vi "Autonomous.vi"() -> ()   [LabVIEW 2017]
doc: "This VI starts when autonomous period begins, and will automatically be terminated when it ends. You can carry out timed or sensor driven operations directly to I/O or to subsystems without needing to return to the caller."
uses:
  Motion_Profiler_Class-master/MotionProfiles.lvclass
  <vilib>/Rock Robotics/WPI/SafetyOutput/WPI_SafetyOutputConfigMenu.ctl
  fa3d0b00-d70b-4d5b-8447-19f35fb7f60c.vi
  d1af4e31-2977-4334-b470-f567b7f2c4f2.vi
  <vilib>/Rock Robotics/Network Tables/NT Read String.vi
  <vilib>/Rock Robotics/WPI/Utilities/WPI_GetSetVariantRefNum.vi
  <vilib>/Rock Robotics/Network Tables/NT Read Boolean.vi
panel:
  out "Left Motor":T1(graph)
  out "Left Throttle":dbl(graph)
  out "Right Motor":T2(graph)
  out "Right Throttle":dbl(graph)
  out "Right Bottom Buf Count":i32
  out "Left Bottom Buf Count":i32
  out "Right Under Run":bool
  out "Left Under Run":bool
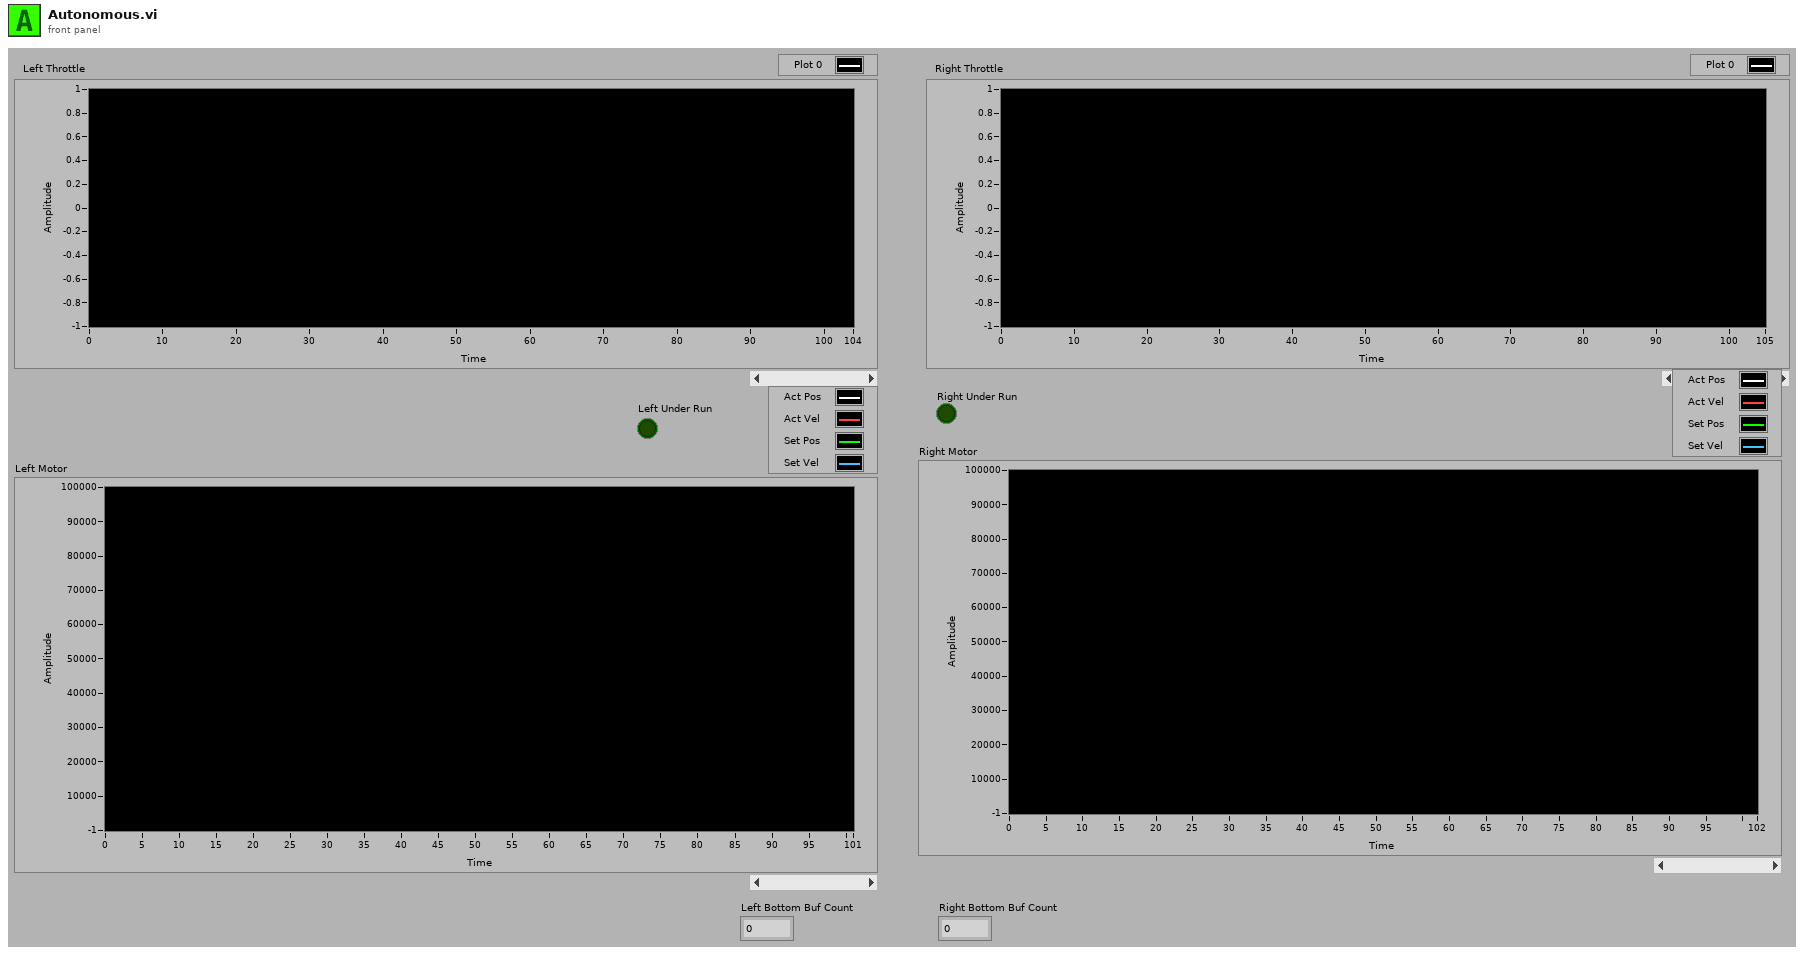
[diagram p1: front panel]
types:
  T1 = cluster{"Set_Pos_(u)":i32, "Set_Pos_(u)":i32, "Act_Vel_(u/100ms)":i32, "Set_Vel_(u/100ms)":i32}
  T2 = cluster{"Set_Vel_(u/100ms)":i32, "Act_Vel_(u/100ms)":i32, "Set_Pos_(u)":i32, "Act_Pos(u)":i32}
  T3 = typedef "WPI_SafetyOutputConfigMenu.ctl" = enum16{"Enable", "Disable"}
  T4 = typedef "WPI_RobotDriveDevRef.ctl" = cluster{"DevStatus":errorcluster, "Motors[]":T5[], "Square Inputs":bool, "Max Output":dbl}
  T5 = typedef "WPI_MotorControlDeviceRef.ctl" = cluster{"DeviceStatus":errorcluster, "Type":T6, "PWM":cluster{"PWM Channel":T7, "DeadBand":T8}, "CAN":cluster{"Device Number":u8, "SetOutput VI Ref":variant, "GetOutput VI Ref":variant, "Enable VI Ref":variant, "Disable VI Ref":variant, "Data":variant}, "Invert":bool, "DIO PWM":cluster{"PWM \"Enable\" Channel":T7, "DIOChannel":T9, "PWM Rate":dbl}}
  T6 = typedef "WPI_MotorControlType.ctl" = enum16{"PWM", "CAN", "DIO PWM"}
  T7 = typedef "FPGA_DIOPWMChannel.ctl" = enum8{"PWM 0", "PWM 1", "PWM 2", "PWM 3", "PWM 4", "PWM 5", "PWM 6", "PWM 7", "PWM 8", "PWM 9", "PWM MXP 0", "PWM MXP 1", "PWM MXP 2", "PWM MXP 3", "PWM MXP 4", "PWM MXP 5", "PWM MXP 6", "PWM MXP 7", "PWM MXP 8", "PWM MXP 9", "Invalid"}
  T8 = typedef "WPI_PWMDeadband.ctl" = cluster{"Name":string, "maxPositivePwm":i32, "minPositivePwm":i32, "centerPwm":i32, "maxNegativePwm":i32, "minNegativePwm":i32, "angularRange":u16}
  T9 = typedef "FPGA_DIOChannel.ctl" = enum8{"DIO 0", "DIO 1", "DIO 2", "DIO 3", "DIO 4", "DIO 5", "DIO 6", "DIO 7", "DIO 8", "DIO 9", "DIO MXP 0", "DIO MXP 1", "DIO MXP 2", "DIO MXP 3", "DIO MXP 4", "DIO MXP 5", "DIO MXP 6", "DIO MXP 7", "DIO MXP 8", "DIO MXP 9", "DIO MXP 10", "DIO MXP 11", "DIO MXP 12", "DIO MXP 13", "DIO MXP 14", "DIO MXP 15", "SPI Port CS1", "SPI Port CS2", "SPI Port CS3", "SPI Port MISO", "SPI Port MOSI", "Invalid"}
  T10 = typedef "MotionProfiles.lvclass/MotionProfile_MP_Class_Status.ctl" = cluster{"Motion Profile Status":cluster{"Top Buffer Remaining":i32, "Top Buffer Count":i32, "Bottom Buffer Count":i32, "Has Underrun?":bool, "Is Underrun?":bool, "Active Point Valid?":bool, "Is Last?":bool, "Profile Slot Select 0":i32, "Output Enable":i32, "Time Duration (ms)":i32, "Profile Slot Select 1":i32}, "TalonState":T11, "MP Is Done":bool, "MP Is Executing":bool, "Set_Vel_(u/100ms)":i32, "Set_Pos_(u)":i32, "Act_Vel_(u/100ms)":i32, "Act_Pos(u)":i32, "Throtle":dbl}
  T11 = typedef "MotionProfiles.lvclass/MotionProfile_TalonSetValueEnum.ctl" = enum16{"Disable", "Enable", "Hold"}
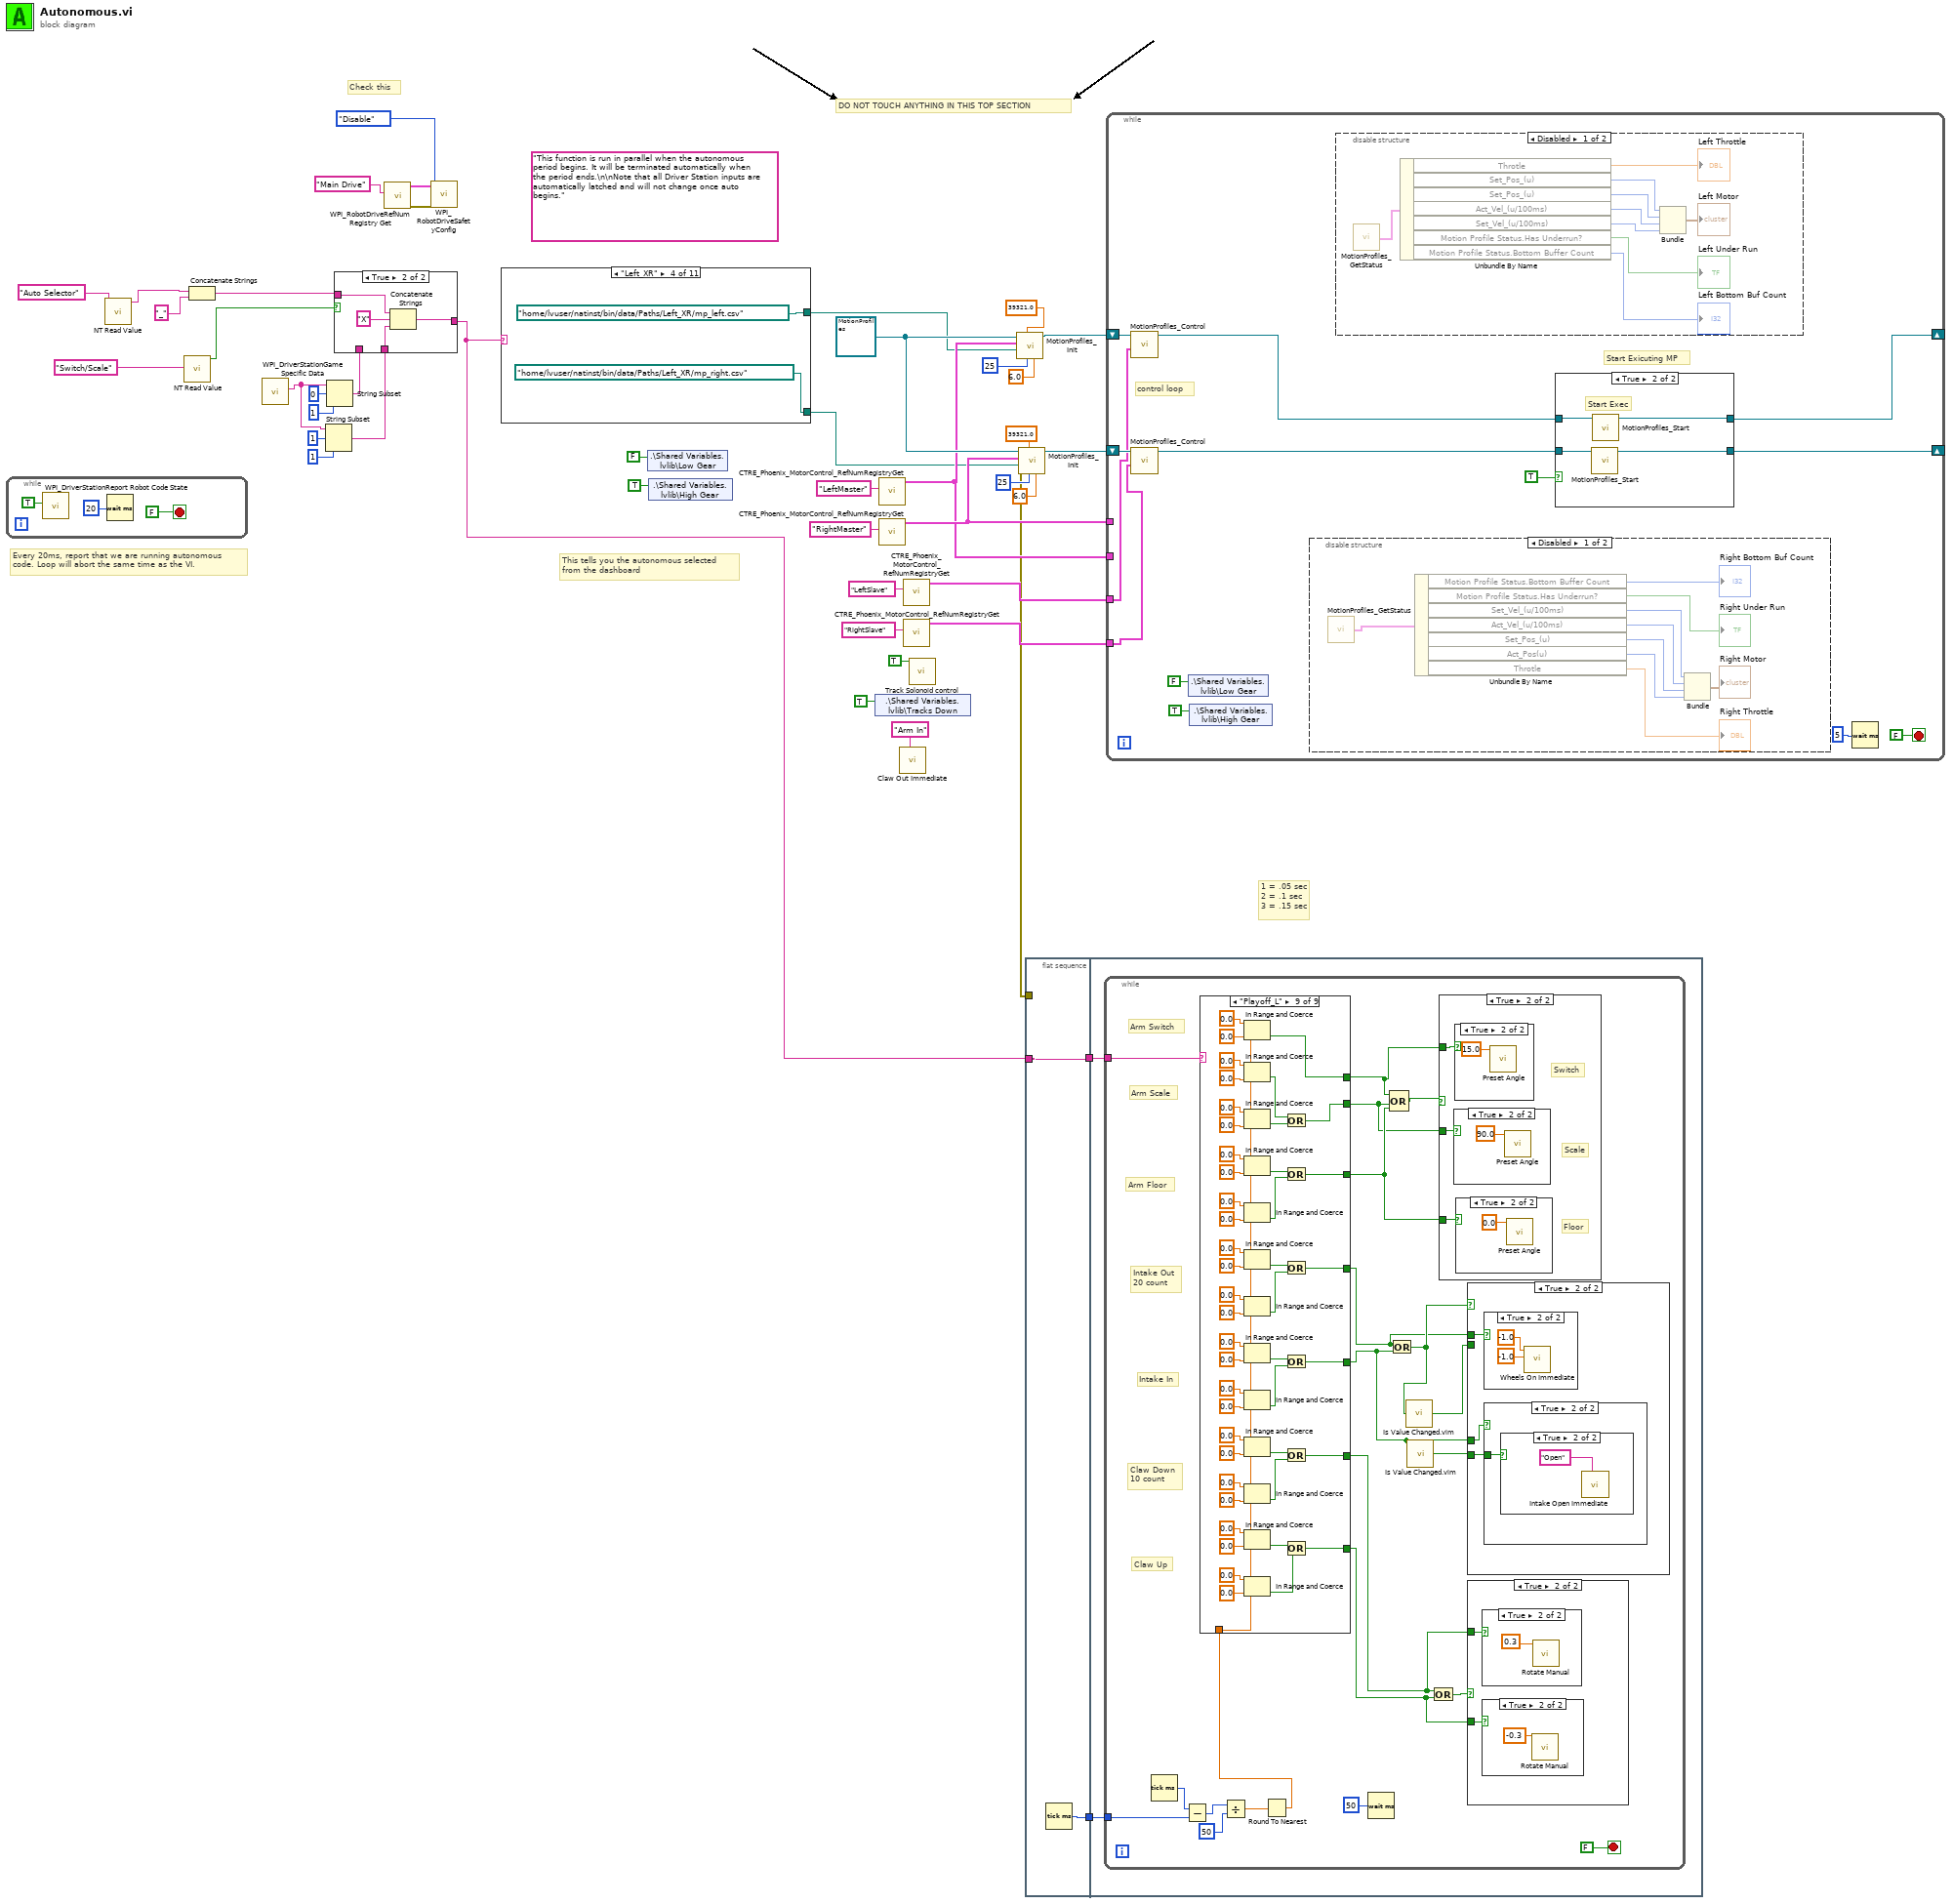
[diagram p0: block diagram]
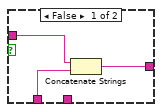
[diagram p2: hidden frame]
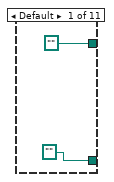
[diagram p3: hidden frame]
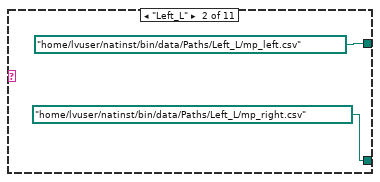
[diagram p4: hidden frame]
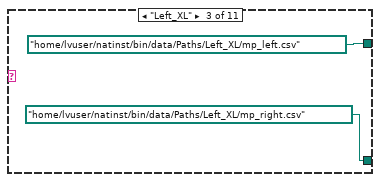
[diagram p5: hidden frame]
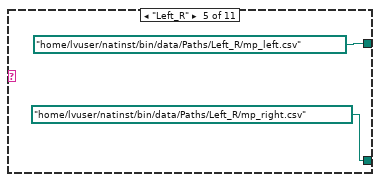
[diagram p6: hidden frame]
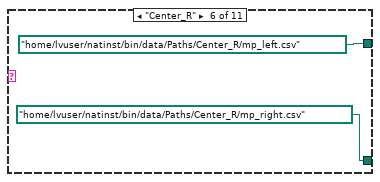
[diagram p7: hidden frame]
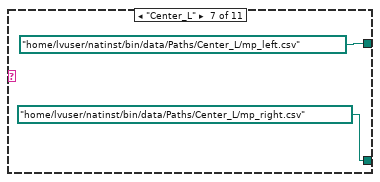
[diagram p8: hidden frame]
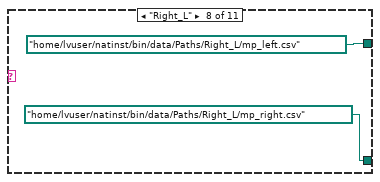
[diagram p9: hidden frame]
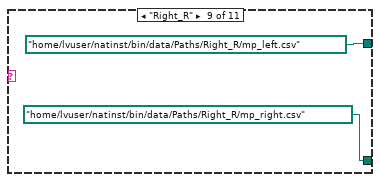
[diagram p10: hidden frame]
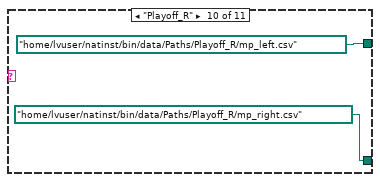
[diagram p11: hidden frame]
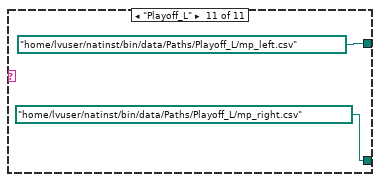
[diagram p12: hidden frame]
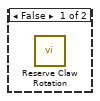
[diagram p13: hidden frame]
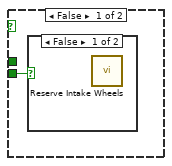
[diagram p16: hidden frame]
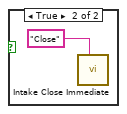
[diagram p17: hidden frame]
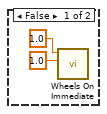
[diagram p20: hidden frame]
diagram:
  w41 = refnum<class "MotionProfiles.lvclass"> refnum ("MotionProfiles.lvclass")
  (unwired) "This function is run in parallel when the autonomous period begins. It will be terminated automatically when the period ends.\n\nNote that all Driver Station inputs are automatically latched and will not change once auto begins."
  # "1 = .05 sec\n2 = .1 sec\n3 = .15 sec"
  # "Check this"
  # "DO NOT TOUCH ANYTHING IN THIS TOP SECTION"
  # "This tells you the autonomous selected\nfrom the dashboard"
  # "Every 20ms, report that we are running autonomous\ncode. Loop will abort the same time as the VI."
  n1 = while {
    stop <- FALSE stop-if-true
    n2 = call <vilib>:"WPI_DriverStationReport Robot Code State.vi"("Autonomous"=TRUE) -> ()  [unwired: 10 in, 1 out]
    n3 = Wait (ms)(milliseconds to wait=u32 20) -> ()  [unwired: 1 out]
  }
  n4 = call-poly <vilib>:"NT Read Value.vi"("Name"="Auto Selector") -> ("String"=w19:string)  [unwired: 9 in, 1 out]
  n5 = call-poly <vilib>:"NT Read Value.vi"("Name"="Switch/Scale") -> ("Boolean"=w2:bool)  [unwired: 9 in, 1 out]
  n6 = Concatenate Strings(w19, "_" ("string")) -> (w6:string)
  n7 = call <vilib>:"WPI_DriverStationGame Specific Data.vi"() -> ("Game Specific Data"=w7:string)  [unwired: 11 in]
  n8 = String Subset(string=w7, offset (0)=1, length (rest)=1 ("length (rest)")) -> (substring=w5:string)
  n9 = String Subset(string=w7, offset (0)=0, length (rest)=1 ("length (rest)")) -> (substring=w4:string)
  n10 = case shown="True" w2 {
    tunnel: w6 -> [w50 w55]
    tunnel: w5 -> [_ w53]
    tunnel: w4 -> [w51 _]
    tunnel: [w49 w52] -> w3
    frame False {
      n11 = Concatenate Strings(w50, w51) -> (w49:string)
    }
    frame True {
      n12 = Concatenate Strings(w55, "X" ("string"), w53) -> (w52:string)
    }
  }
  n13 = call <vilib>:"WPI_RobotDriveRefNum Registry Get.vi"("refnum name"="Main Drive") -> ("error out"=w17:errorcluster, "RobotDriveDevRef"=w16:T4)  [unwired: 9 in]
  n14 = call <vilib>:"WPI_RobotDriveSafetyConfig.vi"("error in (no error)"=w17, "mode"=WPI_SafetyOutputConfigMenu."Disable", "RobotDriveDevRef"=w16) -> ()  [unwired: 7 in, 2 out]
  n15 = case shown="\"Left_XR\"" w3 {
    tunnel: [path "" path "/home/lvuser/natinst/bin/data/Paths/Left_L/mp_right.csv" ("file path (use dialog)") path "/home/lvuser/natinst/bin/data/Paths/Left_XL/mp_right.csv" ("file path (use dialog)") path "/home/lvuser/natinst/bin/data/Paths/Left_XR/mp_right.csv" ("file path (use dialog)") path "/home/lvuser/natinst/bin/data/Paths/Left_R/mp_right.csv" ("file path (use dialog)") path "/home/lvuser/natinst/bin/data/Paths/Center_R/mp_right.csv" ("file path (use dialog)") path "/home/lvuser/natinst/bin/data/Paths/Center_L/mp_right.csv" ("file path (use dialog)") path "/home/lvuser/natinst/bin/data/Paths/Right_L/mp_right.csv" ("file path (use dialog)") path "/home/lvuser/natinst/bin/data/Paths/Right_R/mp_right.csv" ("file path (use dialog)") path "/home/lvuser/natinst/bin/data/Paths/Playoff_R/mp_right.csv" ("file path (use dialog)") path "/home/lvuser/natinst/bin/data/Paths/Playoff_L/mp_right.csv" ("file path (use dialog)")] -> w12
    tunnel: [path "" path "/home/lvuser/natinst/bin/data/Paths/Left_L/mp_left.csv" ("file path (use dialog)") path "/home/lvuser/natinst/bin/data/Paths/Left_XL/mp_left.csv" ("file path (use dialog)") path "/home/lvuser/natinst/bin/data/Paths/Left_XR/mp_left.csv" ("file path (use dialog)") path "/home/lvuser/natinst/bin/data/Paths/Left_R/mp_left.csv" ("file path (use dialog)") path "/home/lvuser/natinst/bin/data/Paths/Center_R/mp_left.csv" ("file path (use dialog)") path "/home/lvuser/natinst/bin/data/Paths/Center_L/mp_left.csv" ("file path (use dialog)") path "/home/lvuser/natinst/bin/data/Paths/Right_L/mp_left.csv" ("file path (use dialog)") path "/home/lvuser/natinst/bin/data/Paths/Right_R/mp_left.csv" ("file path (use dialog)") path "/home/lvuser/natinst/bin/data/Paths/Playoff_R/mp_left.csv" ("file path (use dialog)") path "/home/lvuser/natinst/bin/data/Paths/Playoff_L/mp_left.csv" ("file path (use dialog)")] -> w11
    frame Default {
    }
    frame "Left_L" {
    }
    frame "Left_XL" {
    }
    frame "Left_XR" {
    }
    frame "Left_R" {
    }
    frame "Center_R" {
    }
    frame "Center_L" {
    }
    frame "Right_L" {
    }
    frame "Right_R" {
    }
    frame "Playoff_R" {
    }
    frame "Playoff_L" {
    }
  }
  n16 = shared-variable ".\\Shared Variables.lvlib\\Low Gear"(FALSE ("Low Gear")) -> ()  [unwired: 1 in, 1 out]
  n17 = shared-variable ".\\Shared Variables.lvlib\\High Gear"(TRUE ("High Gear")) -> ()  [unwired: 1 in, 1 out]
  n18 = shared-variable ".\\Shared Variables.lvlib\\Tracks Down"(TRUE ("High Gear")) -> ()  [unwired: 1 in, 1 out]
  n19 = call <vilib>:"CTRE_Phoenix_MotorControl_RefNumRegistryGet.vi"("refnum name"="LeftMaster") -> ("PhoenixMotorControlDevRef"=w32:T5)  [unwired: 9 in, 1 out]
  n20 = call <vilib>:"CTRE_Phoenix_MotorControl_RefNumRegistryGet.vi"("refnum name"="RightMaster") -> ("PhoenixMotorControlDevRef"=w33:T5)  [unwired: 9 in, 1 out]
  n21 = call "Claw Out Immediate.vi"("Description"="Arm In") -> ()  [unwired: 10 in, 1 out]
  n22 = call <vilib>:"CTRE_Phoenix_MotorControl_RefNumRegistryGet.vi"("refnum name"="LeftSlave") -> ("PhoenixMotorControlDevRef"=w26:T5)  [unwired: 9 in, 1 out]
  n23 = call <vilib>:"CTRE_Phoenix_MotorControl_RefNumRegistryGet.vi"("refnum name"="RightSlave") -> ("PhoenixMotorControlDevRef"=w25:T5)  [unwired: 9 in, 1 out]
  n24 = call "Track Solonoid control.vi"("Manual Tracks"=TRUE) -> ()  [unwired: 11 in]
  n25 = call "MotionProfiles_Init.vi"("Wheel_Diameter (in)"=6.0 ("Wheel Diameter"), "MP_Frame_Rate_(ms)"=25, "Encoder_CPR_4x"=39321.0, "CSV File Path"=w11, "PhoenixMotorControlDevRef"=w32, "MotionProfiles in"=w41) -> ("MotionProfiles out"=w44:refnum<class "MotionProfiles.lvclass">)  [unwired: 4 in, 1 out]
  n26 = call "MotionProfiles_Init.vi"("Wheel_Diameter (in)"=6.0, "MP_Frame_Rate_(ms)"=25, "Encoder_CPR_4x"=39321.0, "CSV File Path"=w12, "PhoenixMotorControlDevRef"=w33, "MotionProfiles in"=w41) -> ("error out"=w24:errorcluster, "MotionProfiles out"=w42:refnum<class "MotionProfiles.lvclass">)  [unwired: 4 in]
  n27 = flat-sequence {
    tunnel: [w79] -> w14
    tunnel: [w78] -> w13
    tunnel: w3 -> [w78]
    tunnel: w24 -> [_]
    tunnel: w14 -> [w81]
    tunnel: w13 -> [w80]
    frame #0 {
      n28 = Tick Count (ms)() -> (millisecond timer value=w79:u32)
    }
    frame #1 {
      n29 = while {
        tunnel: w80 -> [w98]
        tunnel: w81 -> [w99]
        stop <- FALSE stop-if-true
        # "Intake In"
        # "Intake Out\n20 count"
        # "Claw Up"
        # "Claw Down\n10 count"
        # "Arm Floor"
        # "Arm Scale"
        # "Arm Switch"
        n30 = Tick Count (ms)() -> (millisecond timer value=w101:u32)
        n31 = Subtract(x=w101, y=w99) -> (x-y=w83:u32)
        n32 = Divide(x=w83, y=u32 50) -> (x/y=w100:dbl)
        n33 = Round To Nearest(number=w100) -> (nearest integer value=w97:dbl)
        n34 = case shown="\"Playoff_L\"" w98 {
          tunnel: w97 -> [_ w132 w178 w224 w270 w316 w362 w408 w454]
          tunnel: [FALSE w173 w219 w265 w311 w357 w403 w449 w495] -> w90
          tunnel: [FALSE w176 w222 w268 w314 w360 w406 w452 w498] -> w85
          tunnel: [FALSE w170 w216 w262 w308 w354 w400 w446 w492] -> w86
          tunnel: [FALSE w167 w213 w259 w305 w351 w397 w443 w489] -> w87
          tunnel: [FALSE w140 w186 w232 w278 w324 w370 w416 w462] -> w89
          tunnel: [FALSE w139 w185 w231 w277 w323 w369 w415 w461] -> w88
          tunnel: [FALSE w131 w177 w223 w269 w315 w361 w407 w453] -> w84
          frame Default {
          }
          frame "Right_R" {
            n35 = In Range and Coerce(upper limit=0.0, x=w132, lower limit=0.0) -> (In Range?=w173:bool)  [unwired: 1 out]
            n36 = In Range and Coerce(upper limit=0.0, x=w132, lower limit=0.0) -> (In Range?=w152:bool)  [unwired: 1 out]
            n37 = In Range and Coerce(upper limit=0.0, x=w132, lower limit=0.0) -> (In Range?=w151:bool)  [unwired: 1 out]
            n38 = In Range and Coerce(upper limit=0.0, x=w132, lower limit=0.0) -> (In Range?=w146:bool)  [unwired: 1 out]
            n39 = In Range and Coerce(upper limit=0.0, x=w132, lower limit=0.0) -> (In Range?=w145:bool)  [unwired: 1 out]
            n40 = In Range and Coerce(upper limit=140.0, x=w132, lower limit=120.0) -> (In Range?=w169:bool)  [unwired: 1 out]
            n41 = In Range and Coerce(upper limit=0.0 ("x"), x=w132, lower limit=0.0) -> (In Range?=w168:bool)  [unwired: 1 out]
            n42 = In Range and Coerce(upper limit=0.0, x=w132, lower limit=0.0) -> (In Range?=w172:bool)  [unwired: 1 out]
            n43 = In Range and Coerce(upper limit=0.0, x=w132, lower limit=0.0) -> (In Range?=w171:bool)  [unwired: 1 out]
            n44 = In Range and Coerce(upper limit=120.0, x=w132, lower limit=110.0) -> (In Range?=w175:bool)  [unwired: 1 out]
            n45 = In Range and Coerce(upper limit=0.0, x=w132, lower limit=0.0) -> (In Range?=w174:bool)  [unwired: 1 out]
            n46 = In Range and Coerce(upper limit=0.0, x=w132, lower limit=0.0) -> (In Range?=w138:bool)  [unwired: 1 out]
            n47 = In Range and Coerce(upper limit=0.0, x=w132, lower limit=0.0) -> (In Range?=w137:bool)  [unwired: 1 out]
            n48 = Or(x=w152, y=w151) -> (x .or. y?=w139:bool)
            n49 = Or(x=w146, y=w145) -> (x .or. y?=w140:bool)
            n50 = Or(x=w169, y=w168) -> (x .or. y?=w167:bool)
            n51 = Or(x=w172, y=w171) -> (x .or. y?=w170:bool)
            n52 = Or(x=w175, y=w174) -> (x .or. y?=w176:bool)
            n53 = Or(x=w138, y=w137) -> (x .or. y?=w131:bool)
          }
          frame "Right_L" {
            n54 = In Range and Coerce(upper limit=0.0, x=w178, lower limit=0.0) -> (In Range?=w219:bool)  [unwired: 1 out]
            n55 = In Range and Coerce(upper limit=0.0, x=w178, lower limit=0.0) -> (In Range?=w198:bool)  [unwired: 1 out]
            n56 = In Range and Coerce(upper limit=0.0, x=w178, lower limit=0.0) -> (In Range?=w197:bool)  [unwired: 1 out]
            n57 = In Range and Coerce(upper limit=0.0, x=w178, lower limit=0.0) -> (In Range?=w192:bool)  [unwired: 1 out]
            n58 = In Range and Coerce(upper limit=0.0, x=w178, lower limit=0.0) -> (In Range?=w191:bool)  [unwired: 1 out]
            n59 = In Range and Coerce(upper limit=270.0, x=w178, lower limit=250.0) -> (In Range?=w215:bool)  [unwired: 1 out]
            n60 = In Range and Coerce(upper limit=0.0 ("x"), x=w178, lower limit=0.0) -> (In Range?=w214:bool)  [unwired: 1 out]
            n61 = In Range and Coerce(upper limit=0.0, x=w178, lower limit=0.0) -> (In Range?=w218:bool)  [unwired: 1 out]
            n62 = In Range and Coerce(upper limit=0.0, x=w178, lower limit=0.0) -> (In Range?=w217:bool)  [unwired: 1 out]
            n63 = In Range and Coerce(upper limit=250.0, x=w178, lower limit=240.0) -> (In Range?=w221:bool)  [unwired: 1 out]
            n64 = In Range and Coerce(upper limit=0.0, x=w178, lower limit=0.0) -> (In Range?=w220:bool)  [unwired: 1 out]
            n65 = In Range and Coerce(upper limit=0.0, x=w178, lower limit=0.0) -> (In Range?=w184:bool)  [unwired: 1 out]
            n66 = In Range and Coerce(upper limit=0.0, x=w178, lower limit=0.0) -> (In Range?=w183:bool)  [unwired: 1 out]
            n67 = Or(x=w198, y=w197) -> (x .or. y?=w185:bool)
            n68 = Or(x=w192, y=w191) -> (x .or. y?=w186:bool)
            n69 = Or(x=w215, y=w214) -> (x .or. y?=w213:bool)
            n70 = Or(x=w218, y=w217) -> (x .or. y?=w216:bool)
            n71 = Or(x=w221, y=w220) -> (x .or. y?=w222:bool)
            n72 = Or(x=w184, y=w183) -> (x .or. y?=w177:bool)
          }
          frame "Left_R" {
            n73 = In Range and Coerce(upper limit=0.0, x=w224, lower limit=0.0) -> (In Range?=w265:bool)  [unwired: 1 out]
            n74 = In Range and Coerce(upper limit=0.0, x=w224, lower limit=0.0) -> (In Range?=w244:bool)  [unwired: 1 out]
            n75 = In Range and Coerce(upper limit=0.0, x=w224, lower limit=0.0) -> (In Range?=w243:bool)  [unwired: 1 out]
            n76 = In Range and Coerce(upper limit=0.0, x=w224, lower limit=0.0) -> (In Range?=w238:bool)  [unwired: 1 out]
            n77 = In Range and Coerce(upper limit=0.0, x=w224, lower limit=0.0) -> (In Range?=w237:bool)  [unwired: 1 out]
            n78 = In Range and Coerce(upper limit=270.0, x=w224, lower limit=250.0) -> (In Range?=w261:bool)  [unwired: 1 out]
            n79 = In Range and Coerce(upper limit=0.0 ("x"), x=w224, lower limit=0.0) -> (In Range?=w260:bool)  [unwired: 1 out]
            n80 = In Range and Coerce(upper limit=0.0, x=w224, lower limit=0.0) -> (In Range?=w264:bool)  [unwired: 1 out]
            n81 = In Range and Coerce(upper limit=0.0, x=w224, lower limit=0.0) -> (In Range?=w263:bool)  [unwired: 1 out]
            n82 = In Range and Coerce(upper limit=250.0, x=w224, lower limit=240.0) -> (In Range?=w267:bool)  [unwired: 1 out]
            n83 = In Range and Coerce(upper limit=0.0, x=w224, lower limit=0.0) -> (In Range?=w266:bool)  [unwired: 1 out]
            n84 = In Range and Coerce(upper limit=0.0, x=w224, lower limit=0.0) -> (In Range?=w230:bool)  [unwired: 1 out]
            n85 = In Range and Coerce(upper limit=0.0, x=w224, lower limit=0.0) -> (In Range?=w229:bool)  [unwired: 1 out]
            n86 = Or(x=w244, y=w243) -> (x .or. y?=w231:bool)
            n87 = Or(x=w238, y=w237) -> (x .or. y?=w232:bool)
            n88 = Or(x=w261, y=w260) -> (x .or. y?=w259:bool)
            n89 = Or(x=w264, y=w263) -> (x .or. y?=w262:bool)
            n90 = Or(x=w267, y=w266) -> (x .or. y?=w268:bool)
            n91 = Or(x=w230, y=w229) -> (x .or. y?=w223:bool)
          }
          frame "Left_L" {
            n92 = In Range and Coerce(upper limit=0.0, x=w270, lower limit=0.0) -> (In Range?=w311:bool)  [unwired: 1 out]
            n93 = In Range and Coerce(upper limit=0.0, x=w270, lower limit=0.0) -> (In Range?=w290:bool)  [unwired: 1 out]
            n94 = In Range and Coerce(upper limit=0.0, x=w270, lower limit=0.0) -> (In Range?=w289:bool)  [unwired: 1 out]
            n95 = In Range and Coerce(upper limit=0.0, x=w270, lower limit=0.0) -> (In Range?=w284:bool)  [unwired: 1 out]
            n96 = In Range and Coerce(upper limit=0.0, x=w270, lower limit=0.0) -> (In Range?=w283:bool)  [unwired: 1 out]
            n97 = In Range and Coerce(upper limit=140.0, x=w270, lower limit=120.0) -> (In Range?=w307:bool)  [unwired: 1 out]
            n98 = In Range and Coerce(upper limit=0.0 ("x"), x=w270, lower limit=0.0) -> (In Range?=w306:bool)  [unwired: 1 out]
            n99 = In Range and Coerce(upper limit=0.0, x=w270, lower limit=0.0) -> (In Range?=w310:bool)  [unwired: 1 out]
            n100 = In Range and Coerce(upper limit=0.0, x=w270, lower limit=0.0) -> (In Range?=w309:bool)  [unwired: 1 out]
            n101 = In Range and Coerce(upper limit=120.0, x=w270, lower limit=110.0) -> (In Range?=w313:bool)  [unwired: 1 out]
            n102 = In Range and Coerce(upper limit=0.0, x=w270, lower limit=0.0) -> (In Range?=w312:bool)  [unwired: 1 out]
            n103 = In Range and Coerce(upper limit=0.0, x=w270, lower limit=0.0) -> (In Range?=w276:bool)  [unwired: 1 out]
            n104 = In Range and Coerce(upper limit=0.0, x=w270, lower limit=0.0) -> (In Range?=w275:bool)  [unwired: 1 out]
            n105 = Or(x=w290, y=w289) -> (x .or. y?=w277:bool)
            n106 = Or(x=w284, y=w283) -> (x .or. y?=w278:bool)
            n107 = Or(x=w307, y=w306) -> (x .or. y?=w305:bool)
            n108 = Or(x=w310, y=w309) -> (x .or. y?=w308:bool)
            n109 = Or(x=w313, y=w312) -> (x .or. y?=w314:bool)
            n110 = Or(x=w276, y=w275) -> (x .or. y?=w269:bool)
          }
          frame "Center_L" {
            n111 = In Range and Coerce(upper limit=0.0, x=w316, lower limit=0.0) -> (In Range?=w357:bool)  [unwired: 1 out]
            n112 = In Range and Coerce(upper limit=0.0, x=w316, lower limit=0.0) -> (In Range?=w336:bool)  [unwired: 1 out]
            n113 = In Range and Coerce(upper limit=0.0, x=w316, lower limit=0.0) -> (In Range?=w335:bool)  [unwired: 1 out]
            n114 = In Range and Coerce(upper limit=0.0, x=w316, lower limit=0.0) -> (In Range?=w330:bool)  [unwired: 1 out]
            n115 = In Range and Coerce(upper limit=0.0, x=w316, lower limit=0.0) -> (In Range?=w329:bool)  [unwired: 1 out]
            n116 = In Range and Coerce(upper limit=110.0, x=w316, lower limit=100.0) -> (In Range?=w353:bool)  [unwired: 1 out]
            n117 = In Range and Coerce(upper limit=0.0 ("x"), x=w316, lower limit=0.0) -> (In Range?=w352:bool)  [unwired: 1 out]
            n118 = In Range and Coerce(upper limit=0.0, x=w316, lower limit=0.0) -> (In Range?=w356:bool)  [unwired: 1 out]
            n119 = In Range and Coerce(upper limit=0.0, x=w316, lower limit=0.0) -> (In Range?=w355:bool)  [unwired: 1 out]
            n120 = In Range and Coerce(upper limit=100.0, x=w316, lower limit=90.0) -> (In Range?=w359:bool)  [unwired: 1 out]
            n121 = In Range and Coerce(upper limit=0.0, x=w316, lower limit=0.0) -> (In Range?=w358:bool)  [unwired: 1 out]
            n122 = In Range and Coerce(upper limit=0.0, x=w316, lower limit=0.0) -> (In Range?=w322:bool)  [unwired: 1 out]
            n123 = In Range and Coerce(upper limit=0.0, x=w316, lower limit=0.0) -> (In Range?=w321:bool)  [unwired: 1 out]
            n124 = Or(x=w336, y=w335) -> (x .or. y?=w323:bool)
            n125 = Or(x=w330, y=w329) -> (x .or. y?=w324:bool)
            n126 = Or(x=w353, y=w352) -> (x .or. y?=w351:bool)
            n127 = Or(x=w356, y=w355) -> (x .or. y?=w354:bool)
            n128 = Or(x=w359, y=w358) -> (x .or. y?=w360:bool)
            n129 = Or(x=w322, y=w321) -> (x .or. y?=w315:bool)
          }
          frame "Center_R" {
            n130 = In Range and Coerce(upper limit=0.0, x=w362, lower limit=0.0) -> (In Range?=w403:bool)  [unwired: 1 out]
            n131 = In Range and Coerce(upper limit=0.0, x=w362, lower limit=0.0) -> (In Range?=w382:bool)  [unwired: 1 out]
            n132 = In Range and Coerce(upper limit=0.0, x=w362, lower limit=0.0) -> (In Range?=w381:bool)  [unwired: 1 out]
            n133 = In Range and Coerce(upper limit=0.0, x=w362, lower limit=0.0) -> (In Range?=w376:bool)  [unwired: 1 out]
            n134 = In Range and Coerce(upper limit=0.0, x=w362, lower limit=0.0) -> (In Range?=w375:bool)  [unwired: 1 out]
            n135 = In Range and Coerce(upper limit=120.0, x=w362, lower limit=100.0) -> (In Range?=w399:bool)  [unwired: 1 out]
            n136 = In Range and Coerce(upper limit=0.0 ("x"), x=w362, lower limit=0.0) -> (In Range?=w398:bool)  [unwired: 1 out]
            n137 = In Range and Coerce(upper limit=0.0, x=w362, lower limit=0.0) -> (In Range?=w402:bool)  [unwired: 1 out]
            n138 = In Range and Coerce(upper limit=0.0, x=w362, lower limit=0.0) -> (In Range?=w401:bool)  [unwired: 1 out]
            n139 = In Range and Coerce(upper limit=100.0, x=w362, lower limit=90.0) -> (In Range?=w405:bool)  [unwired: 1 out]
            n140 = In Range and Coerce(upper limit=0.0, x=w362, lower limit=0.0) -> (In Range?=w404:bool)  [unwired: 1 out]
            n141 = In Range and Coerce(upper limit=0.0, x=w362, lower limit=0.0) -> (In Range?=w368:bool)  [unwired: 1 out]
            n142 = In Range and Coerce(upper limit=0.0, x=w362, lower limit=0.0) -> (In Range?=w367:bool)  [unwired: 1 out]
            n143 = Or(x=w382, y=w381) -> (x .or. y?=w369:bool)
            n144 = Or(x=w376, y=w375) -> (x .or. y?=w370:bool)
            n145 = Or(x=w399, y=w398) -> (x .or. y?=w397:bool)
            n146 = Or(x=w402, y=w401) -> (x .or. y?=w400:bool)
            n147 = Or(x=w405, y=w404) -> (x .or. y?=w406:bool)
            n148 = Or(x=w368, y=w367) -> (x .or. y?=w361:bool)
          }
          frame "Playoff_R" {
            n149 = In Range and Coerce(upper limit=0.0, x=w408, lower limit=0.0) -> (In Range?=w449:bool)  [unwired: 1 out]
            n150 = In Range and Coerce(upper limit=0.0, x=w408, lower limit=0.0) -> (In Range?=w428:bool)  [unwired: 1 out]
            n151 = In Range and Coerce(upper limit=0.0, x=w408, lower limit=0.0) -> (In Range?=w427:bool)  [unwired: 1 out]
            n152 = In Range and Coerce(upper limit=0.0, x=w408, lower limit=0.0) -> (In Range?=w422:bool)  [unwired: 1 out]
            n153 = In Range and Coerce(upper limit=0.0, x=w408, lower limit=0.0) -> (In Range?=w421:bool)  [unwired: 1 out]
            n154 = In Range and Coerce(upper limit=0.0, x=w408, lower limit=0.0) -> (In Range?=w445:bool)  [unwired: 1 out]
            n155 = In Range and Coerce(upper limit=0.0 ("x"), x=w408, lower limit=0.0) -> (In Range?=w444:bool)  [unwired: 1 out]
            n156 = In Range and Coerce(upper limit=0.0, x=w408, lower limit=0.0) -> (In Range?=w448:bool)  [unwired: 1 out]
            n157 = In Range and Coerce(upper limit=0.0, x=w408, lower limit=0.0) -> (In Range?=w447:bool)  [unwired: 1 out]
            n158 = In Range and Coerce(upper limit=0.0, x=w408, lower limit=0.0) -> (In Range?=w451:bool)  [unwired: 1 out]
            n159 = In Range and Coerce(upper limit=0.0, x=w408, lower limit=0.0) -> (In Range?=w450:bool)  [unwired: 1 out]
            n160 = In Range and Coerce(upper limit=0.0, x=w408, lower limit=0.0) -> (In Range?=w414:bool)  [unwired: 1 out]
            n161 = In Range and Coerce(upper limit=0.0, x=w408, lower limit=0.0) -> (In Range?=w413:bool)  [unwired: 1 out]
            n162 = Or(x=w428, y=w427) -> (x .or. y?=w415:bool)
            n163 = Or(x=w422, y=w421) -> (x .or. y?=w416:bool)
            n164 = Or(x=w445, y=w444) -> (x .or. y?=w443:bool)
            n165 = Or(x=w448, y=w447) -> (x .or. y?=w446:bool)
            n166 = Or(x=w451, y=w450) -> (x .or. y?=w452:bool)
            n167 = Or(x=w414, y=w413) -> (x .or. y?=w407:bool)
          }
          frame "Playoff_L" {
            n168 = In Range and Coerce(upper limit=0.0, x=w454, lower limit=0.0) -> (In Range?=w495:bool)  [unwired: 1 out]
            n169 = In Range and Coerce(upper limit=0.0, x=w454, lower limit=0.0) -> (In Range?=w474:bool)  [unwired: 1 out]
            n170 = In Range and Coerce(upper limit=0.0, x=w454, lower limit=0.0) -> (In Range?=w473:bool)  [unwired: 1 out]
            n171 = In Range and Coerce(upper limit=0.0, x=w454, lower limit=0.0) -> (In Range?=w468:bool)  [unwired: 1 out]
            n172 = In Range and Coerce(upper limit=0.0, x=w454, lower limit=0.0) -> (In Range?=w467:bool)  [unwired: 1 out]
            n173 = In Range and Coerce(upper limit=0.0, x=w454, lower limit=0.0) -> (In Range?=w491:bool)  [unwired: 1 out]
            n174 = In Range and Coerce(upper limit=0.0 ("x"), x=w454, lower limit=0.0) -> (In Range?=w490:bool)  [unwired: 1 out]
            n175 = In Range and Coerce(upper limit=0.0, x=w454, lower limit=0.0) -> (In Range?=w494:bool)  [unwired: 1 out]
            n176 = In Range and Coerce(upper limit=0.0, x=w454, lower limit=0.0) -> (In Range?=w493:bool)  [unwired: 1 out]
            n177 = In Range and Coerce(upper limit=0.0, x=w454, lower limit=0.0) -> (In Range?=w497:bool)  [unwired: 1 out]
            n178 = In Range and Coerce(upper limit=0.0, x=w454, lower limit=0.0) -> (In Range?=w496:bool)  [unwired: 1 out]
            n179 = In Range and Coerce(upper limit=0.0, x=w454, lower limit=0.0) -> (In Range?=w460:bool)  [unwired: 1 out]
            n180 = In Range and Coerce(upper limit=0.0, x=w454, lower limit=0.0) -> (In Range?=w459:bool)  [unwired: 1 out]
            n181 = Or(x=w474, y=w473) -> (x .or. y?=w461:bool)
            n182 = Or(x=w468, y=w467) -> (x .or. y?=w462:bool)
            n183 = Or(x=w491, y=w490) -> (x .or. y?=w489:bool)
            n184 = Or(x=w494, y=w493) -> (x .or. y?=w492:bool)
            n185 = Or(x=w497, y=w496) -> (x .or. y?=w498:bool)
            n186 = Or(x=w460, y=w459) -> (x .or. y?=w453:bool)
          }
        }
        n187 = Wait (ms)(milliseconds to wait=u32 50) -> ()  [unwired: 1 out]
        n188 = Or(x=w87, y=w86) -> (x .or. y?=w95:bool)
        n189 = Compound Arithmetic op=OR(w90, w88, w89) -> (w91:bool)
        n190 = call "Is Value Changed.vim"("value"=w95) -> ("changed or first call?"=w94:bool)
        n191 = call "Is Value Changed.vim"("value"=w86) -> ("changed or first call?"=w96:bool)
        n192 = Or(x=w85, y=w84) -> (x .or. y?=w92:bool)
        n193 = case shown="True" w91 {
          tunnel: w90 -> [_ w120]
          tunnel: w89 -> [_ w119]
          tunnel: w88 -> [_ w118]
          frame False {
            n194 = call "Reserve Arm Actuator.vi"() -> ()  [unwired: 11 in, 1 out]
          }
          frame True {
            # "Switch"
            # "Scale"
            # "Floor"
            n195 = case shown="True" w118 {
              frame False {
              }
              frame True {
                n196 = call "Preset Angle.vi"("Setpoint"=90.0) -> ()  [unwired: 10 in, 1 out]
              }
            }
            n197 = case shown="True" w120 {
              frame False {
              }
              frame True {
                n198 = call "Preset Angle.vi"("Setpoint"=15.0) -> ()  [unwired: 10 in, 1 out]
              }
            }
            n199 = case shown="True" w119 {
              frame False {
              }
              frame True {
                n200 = call "Preset Angle.vi"("Setpoint"=0.0) -> ()  [unwired: 10 in, 1 out]
              }
            }
          }
        }
        n201 = case shown="True" w92 {
          tunnel: w85 -> [_ w104]
          tunnel: w84 -> [_ w103]
          frame False {
            n202 = call "Reserve Claw Rotation.vi"() -> ()  [unwired: 11 in, 1 out]
          }
          frame True {
            n203 = case shown="True" w104 {
              frame False {
              }
              frame True {
                n204 = call "Rotate Manual.vi"("Setpoint"=0.3) -> ()  [unwired: 10 in, 1 out]
              }
            }
            n205 = case shown="True" w103 {
              frame False {
              }
              frame True {
                n206 = call "Rotate Manual.vi"("Setpoint"=-0.3) -> ()  [unwired: 10 in, 1 out]
              }
            }
          }
        }
        n207 = case shown="True" w95 {
          tunnel: w96 -> [_ w111]
          tunnel: w94 -> [w107 _]
          tunnel: w87 -> [_ w110]
          tunnel: w86 -> [_ w109]
          frame False {
            n208 = case shown="False" w107 {
              frame False {
                n209 = call "Reserve Intake Wheels.vi"() -> ()  [unwired: 11 in, 1 out]
              }
              frame True {
                n210 = call "Intake Close Immediate.vi"("Description"="Close") -> ()  [unwired: 10 in, 1 out]
              }
            }
          }
          frame True {
            n211 = case shown="True" w110 {
              frame False {
              }
              frame True {
                n212 = call "Wheels On Immediate.vi"("Right Wheel"=-1.0, "Left Wheel"=-1.0) -> ()  [unwired: 9 in, 1 out]
              }
            }
            n213 = case shown="True" w109 {
              tunnel: w111 -> [_ w114]
              frame False {
              }
              frame True {
                n214 = case shown="True" w114 {
                  frame False {
                    n215 = call "Wheels On Immediate.vi"("Right Wheel"=1.0, "Left Wheel"=1.0) -> ()  [unwired: 9 in, 1 out]
                  }
                  frame True {
                    n216 = call "Intake Open Immediate.vi"("Description"="Open") -> ()  [unwired: 10 in, 1 out]
                  }
                }
              }
            }
          }
        }
      }
    }
  }
  n217 = while {
    shift-right: [w506] -> _
    shift-left: w44 -> [w509]
    shift-right: [w507] -> _
    shift-left: w42 -> [w508]
    tunnel: w33 -> [_]
    tunnel: w32 -> [_]
    tunnel: w26 -> [w504]
    tunnel: w25 -> [w503]
    stop <- FALSE stop-if-true
    # "control loop"
    # "Start Exicuting MP"
    n218 = call "MotionProfiles_Control.vi"("PhoenixMotorControlDevRef Slave"=w504, "MotionProfiles in"=w509) -> ("MotionProfiles out"=w499:refnum<class "MotionProfiles.lvclass">)  [unwired: 8 in, 1 out]
    n219 = call "MotionProfiles_Control.vi"("PhoenixMotorControlDevRef Slave"=w503, "MotionProfiles in"=w508) -> ("MotionProfiles out"=w500:refnum<class "MotionProfiles.lvclass">)  [unwired: 8 in, 1 out]
    n220 = shared-variable ".\\Shared Variables.lvlib\\Low Gear"(FALSE ("Low Gear")) -> ()  [unwired: 1 in, 1 out]
    n221 = shared-variable ".\\Shared Variables.lvlib\\High Gear"(TRUE ("High Gear")) -> ()  [unwired: 1 in, 1 out]
    n222 = disable-structure shown="Disabled" {
      frame Disabled {
        n223 = call "MotionProfiles_GetStatus.vi"() -> ("MP_Class_Status"=w520:T10)  [unwired: 13 in, 2 out]
        n224 = Unbundle By Name(w520) -> ("Motion Profile Status.Bottom Buffer Count"=→"Right Bottom Buf Count":i32, "Motion Profile Status.Has Underrun?"=→"Right Under Run":bool, "Set_Vel_(u/100ms)"=w516:i32, "Act_Vel_(u/100ms)"=w515:i32, "Set_Pos_(u)"=w514:i32, "Act_Pos(u)"=w513:i32, "Throtle"=→"Right Throttle":dbl)
        n225 = Bundle("Set_Vel_(u/100ms)"=w516, "Act_Vel_(u/100ms)"=w515, "Set_Pos_(u)"=w514, "Act_Pos(u)"=w513) -> (→"Right Motor":T2)  [unwired: 1 in]
      }
      frame Enabled {
      }
    }
    n226 = disable-structure shown="Disabled" {
      frame Disabled {
        n227 = call "MotionProfiles_GetStatus.vi"() -> ("MP_Class_Status"=w529:T10)  [unwired: 13 in, 2 out]
        n228 = Unbundle By Name(w529) -> ("Throtle"=→"Left Throttle":dbl, "Set_Pos_(u)"=w522:i32, "Set_Pos_(u)"=w523:i32, "Act_Vel_(u/100ms)"=w524:i32, "Set_Vel_(u/100ms)"=w525:i32, "Motion Profile Status.Has Underrun?"=→"Left Under Run":bool, "Motion Profile Status.Bottom Buffer Count"=→"Left Bottom Buf Count":i32)
        n229 = Bundle("Set_Pos_(u)"=w522, "Set_Pos_(u)"=w523, "Act_Vel_(u/100ms)"=w524, "Set_Vel_(u/100ms)"=w525) -> (→"Left Motor":T1)  [unwired: 1 in]
      }
      frame Enabled {
      }
    }
    n230 = case shown="True" TRUE {
      tunnel: w499 -> [w531 w535]
      tunnel: w500 -> [w530 w533]
      tunnel: [w530 w532] -> w507
      tunnel: [w531 w534] -> w506
      frame False {
      }
      frame True {
        # "Start Exec"
        n231 = call "MotionProfiles_Start.vi"("MotionProfiles in"=w533) -> ("MotionProfiles out"=w532:refnum<class "MotionProfiles.lvclass">)  [unwired: 9 in, 1 out]
        n232 = call "MotionProfiles_Start.vi"("MotionProfiles in"=w535) -> ("MotionProfiles out"=w534:refnum<class "MotionProfiles.lvclass">)  [unwired: 9 in, 1 out]
      }
    }
    n233 = Wait (ms)(milliseconds to wait=u32 5) -> ()  [unwired: 1 out]
  }
